vi "BLM MoveAndWait.vi"(4 "Mode IS:":bool, 5 "Steps/rot":dbl=8000.0, 6 "error in (no error)":errorcluster, 7 "Position / Distance":dbl=1.0 min=-193273528.32 max=193273528.0 step=0.09 format="%.2f", 8 "Motor Address":string="0", 9 "Instrument Address":refnum<visa-resource-name>) -> (0 "error out":errorcluster, 3 "PORT Address 2":refnum<visa-resource-name>)   [LabVIEW 2025]
doc: "Author: Scott Hannahs <sth@magnet.fsu.edu>\n\nThis software is licensed for use under the “MIT License\"\nCopyright (c) 2025 Scott Hannahs, sth@sth@magnet.sthnet.net\n\nPermission is hereby granted, free of charge, to any person obtaining a copy of this software and associated documentation files (the \"Software\"), to deal in the Software without restriction, including without limitation the rights to use, copy, modify, merge, publish, distribute, sublicense, and/or sell copies of the Software, and to permit persons to whom the Software is furnished to do so, subject to the following conditions: The above copyright notice and this permission notice shall be included in all copies or substantial portions of the Software.\n\nTHE SOFTWARE IS PROVIDED \"AS IS\", WITHOUT WARRANTY OF ANY KIND, EXPRESS OR IMPLIED, INCLUDING BUT NOT LIMITED TO THE WARRANTIES OF MERCHANTABILITY, FITNESS FOR A PARTICULAR PURPOSE AND NONINFRINGEMENT. IN NO EVENT SHALL THE AUTHORS OR COPYRIGHT HOLDERS BE LIABLE FOR ANY CLAIM, DAMAGES OR OTHER LIABILITY, WHETHER IN AN ACTION OF CONTRACT, TORT OR OTHERWISE, ARISING FROM, OUT OF OR IN CONNECTION WITH THE SOFTWARE OR THE USE OR OTHER DEALINGS IN THE SOFTWARE."
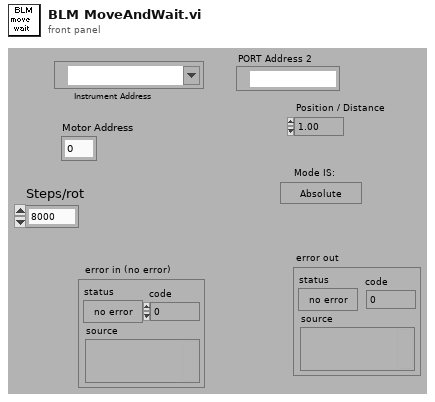
[diagram p1: front panel]
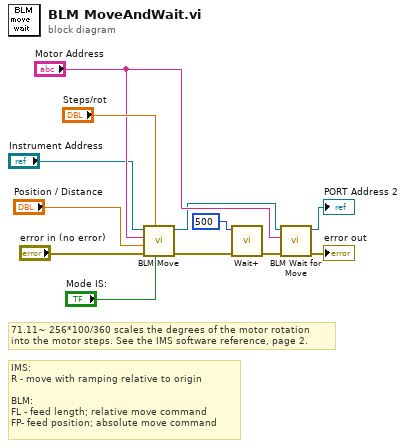
[diagram p0: block diagram]
diagram:
  # "IMS:\nR - move with ramping relative to origin\n\nBLM:\nFL - feed length; relative move command\nFP- feed position; absolute move command"
  # "71.11~ 256*100/360 scales the degrees of the motor rotation\ninto the motor steps. See the IMS software reference, page 2."
  n1 = call "BLM Move.vi"("Mode IS:"="Mode IS:", "Steps/rot"="Steps/rot", "error in (no error)"="error in (no error)", "Position / Distance"="Position / Distance", "Motor Address"="Motor Address", "Port Address"="Instrument Address") -> ("error out"=w12:errorcluster, "Port Address Out"=w2:refnum<visa-resource-name>)  [unwired: 2 in]
  n2 = call "Wait+.vi"("Error In"=w12, "milliseconds to wait"=u32 500) -> ("Error Out"=w11:errorcluster)  [unwired: 4 in, 1 out]
  n3 = call "BLM Wait for Move.vi"("error in (no error)"=w11, "Motor Address"="Motor Address", "PORT Address"=w2) -> ("error out"=→"error out":errorcluster, "PORT Address 2"=→"PORT Address 2":refnum<visa-resource-name>)  [unwired: 3 in, 1 out]
